vi "Add New Line.vi"(8 "error in":errorcluster, 11 "Object Refs":T1) -> (0 "error out":errorcluster, 1 "Success":bool, 2 "Object Refs  out":T1)   [LabVIEW 2015, in "Modbus Module editor node.lvclass"]
uses:
  Modbus Module editor node.lvclass
  <vilib>/NI/DCAF/Tag Editor Core/Table API/Table Manager/object ref.ctl
  <vilib>/NI/DCAF/Tag Editor Core/Configuration Editor/Classes/Engine Parent/Engine Parent Editor Node.lvclass
  <vilib>/NI/DCAF/Tag Editor Core/Configuration Editor/Classes/Module editor node/module editor node.lvclass
  module/configuration/Modbus Module configuration.lvclass
  <vilib>/NI/Tag Bus/tag/tag descriptor.lvclass/tag descriptor.ctl
  <vilib>/NI/Configuration Framework/serializable configuration/NISE_CEF_serializable configuration.lvclass/NISE_CEF_serializable configuration.ctl
  <vilib>/Utility/LVClass/Get LV Class Name.vi
  <vilib>/NI/Configuration Framework/error generator/NISE_error generator.vi
  <vilib>/NI/Module Execution Interface/Engine Configuration/engine configuration.lvclass
  <vilib>/NI/Tag Bus/tag/tag descriptor.lvclass
  <vilib>/NI/Configuration Framework/serializable configuration/NISE_CEF_serializable configuration.lvclass
  <vilib>/NI/DCAF/Tag Editor Core/Table API/Table Manager/Table Manager.lvclass
panel:
  in  "specific class reference":refnum<class "Modbus Module configuration.lvclass">
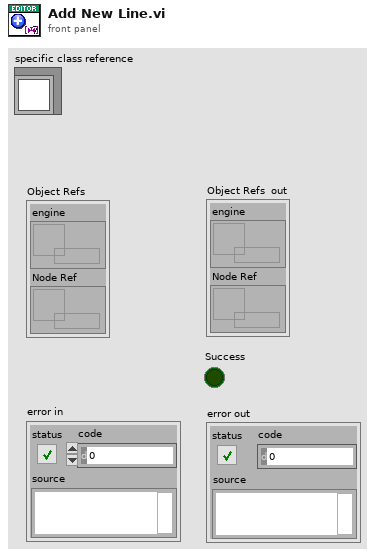
[diagram p1: front panel]
types:
  T1 = typedef "Table Manager.lvlib/Table Manager.lvclass/object ref.ctl" = cluster{"engine":refnum<data-value>, "Node Ref":refnum<data-value>}
  T2 = typedef "Modbus Module editor node.lvclass/table line.ctl" = cluster{"mbchan":refnum<class "Modbus Module Channel.lvclass">, "tag name":string}
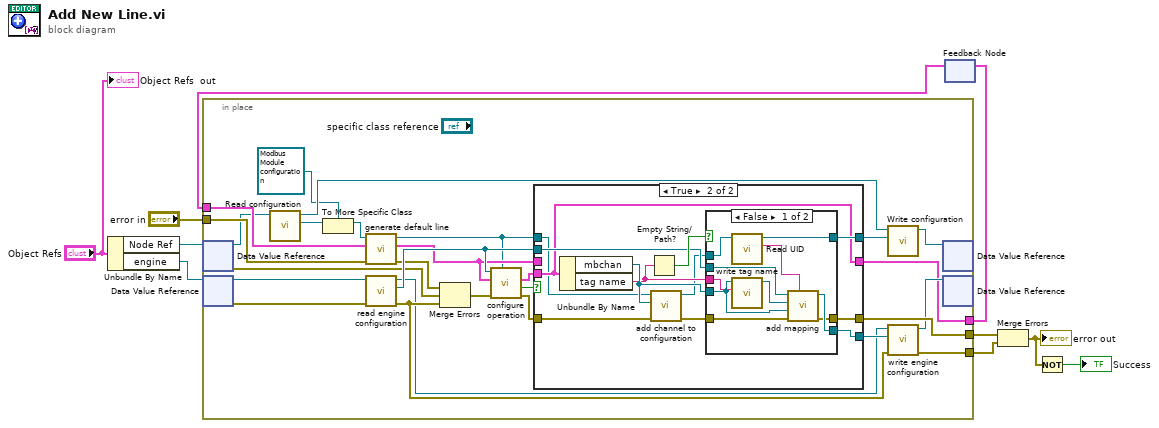
[diagram p0: block diagram]
diagram:
  n1 = Unbundle By Name("Object Refs") -> ("Node Ref"=w6:refnum<data-value>, "engine"=w7:refnum<data-value>)
  n2 = feedback #1() -> (w5:T2)  [unwired: 1 in]
  n3 = in-place {
    in-place-border: [w37] -> w8
    in-place-border: "error in" -> [w20]
    in-place-border: [w25] -> w9
    in-place-border: [w23] -> w10
    in-place-border: w5 -> [w21]
    n4 = in-place-dvr #2(w6) -> (w18:refnum<class "module editor node.lvclass">, w24:errorcluster)
    n5 = in-place-dvr #3(w7) -> (w32:refnum<class "Engine Parent Editor Node.lvclass">, w31:errorcluster)
    n6 = call-dynamic "Read configuration.vi"("NISE_CEF_serializable node in"=w18) -> ("configuration"=w13:refnum<class "NISE_CEF_serializable configuration.lvclass">, "NISE_CEF_serializable node out"=w17:refnum<class "module editor node.lvclass">)  [unwired: 8 in, 1 out]
    n7 = To More Specific Class(target class=refnum<class "Modbus Module configuration.lvclass"> refnum ("Modbus Slave configuration in"), reference=w13) -> (specific class reference=w12:refnum<class "Modbus Module configuration.lvclass">)  [unwired: 1 in, 1 out]
    n8 = call "generate default line.vi"("error in"=w20, "last line"=w21, "Mb Config"=w12) -> ("error out"=w19:errorcluster, "line"=w22:T2, "Modbus Slave configuration out"=w11:refnum<class "Modbus Module configuration.lvclass">)  [unwired: 6 in]
    n9 = call <vilib>:"read engine configuration.vi"("error in"=w31, "Engine Parent Editor Node in"=w32) -> ("error out"=w27:errorcluster, "engine configuration"=w30:refnum<class "engine configuration.lvclass">, "Engine Parent Editor Node out"=w26:refnum<class "Engine Parent Editor Node.lvclass">)  [unwired: 7 in]
    n10 = Merge Errors(w19, w24, w27) -> (w33:errorcluster)
    n11 = call "configure operation.vi"("tag bus configurable plugin module configuration"=w11, "error in"=w33, "line item in"=w22, "engine configuration"=w30) -> ("error out"=w35:errorcluster, "success"=w34:bool, "line item out"=w36:T2)  [unwired: 4 in, 1 out]
    n12 = case shown="True" w34 {
      tunnel: [w41 w44] -> w37
      tunnel: w35 -> [w41 w53]
      tunnel: w30 -> [w40 w51]
      tunnel: w36 -> [_ w43]
      tunnel: [w40 w50] -> w28
      tunnel: [w38 w45] -> w15
      tunnel: w22 -> [w39 _]
      tunnel: [w39 w43] -> w23
      tunnel: w11 -> [w38 w42]
      frame False {
      }
      frame True {
        n13 = Unbundle By Name(w43) -> ("mbchan"=w48:refnum<class "Modbus Module Channel.lvclass">, "tag name"=w47:string)
        n14 = Empty String/Path?(string/path=w47) -> (empty?=w52:bool)
        n15 = call "add channel to configuration.vi"("error in"=w53, "Modbus Module Channel.lvclass"=w48, "Modbus Slave configuration in"=w42) -> ("error out"=w49:errorcluster, "Modbus Slave configuration out"=w46:refnum<class "Modbus Module configuration.lvclass">)  [unwired: 7 in]
        n16 = case shown="False" w52 {
          tunnel: w51 -> [w63 w66]
          tunnel: [w62 w66] -> w50
          tunnel: w49 -> [w61 w65]
          tunnel: w48 -> [w58 _]
          tunnel: w47 -> [w56 _]
          tunnel: [w60 w65] -> w44
          tunnel: w46 -> [w59 w64]
          tunnel: [w55 w64] -> w45
          frame False {
            n17 = call <vilib>:"Read UID.vi"("configuration in"=w59) -> ("instance id"=w54:string, "configuration out"=w55:refnum<class "Modbus Module configuration.lvclass">)  [unwired: 8 in, 1 out]
            n18 = call <vilib>:"write tag name.vi"("name"=w56, "system tag in"=w58) -> ("system tag out"=w57:refnum<class "Modbus Module Channel.lvclass">)  [unwired: 8 in, 1 out]
            n19 = call-dynamic "add mapping.vi"("owner ID"=w54, "error in"=w61, "channel"=w58, "tag descriptor"=w57, "engine configuration"=w63) -> ("error out"=w60:errorcluster, "engine configuration out"=w62:refnum<class "engine configuration.lvclass">)  [unwired: 5 in]
          }
          frame True {
          }
        }
      }
    }
    n20 = call-dynamic "Write configuration.vi"("configuration"=w15, "NISE_CEF_serializable node in"=w17) -> ("NISE_CEF_serializable node out"=w16:refnum<class "module editor node.lvclass">)  [unwired: 8 in, 1 out]
    n21 = call <vilib>:"write engine configuration.vi"("error in"=w27, "engine configuration"=w28, "Engine Parent Editor Node in"=w26) -> ("error out"=w25:errorcluster, "Engine Parent Editor Node out"=w29:refnum<class "Engine Parent Editor Node.lvclass">)  [unwired: 7 in]
    n22 = in-place-dvr #2(w16) -> ()  [unwired: 2 out]
    n23 = in-place-dvr #3(w29) -> ()  [unwired: 2 out]
  }
  n24 = feedback-in #1(w10) -> ()
  n25 = Merge Errors(w8, w9) -> (w2:errorcluster)
  "error out" <- w2
  n26 = Not(x=w2) -> (.not. x?=→"Success":bool)
  "Object Refs  out" <- "Object Refs"
